vi "climber_globals.vi"() -> ()   [LabVIEW 2020]
panel:
  in  "Climber Traversal Piston Command":bool
  out "Climber Lower Command":bool
  out "Climber Raise Command":bool
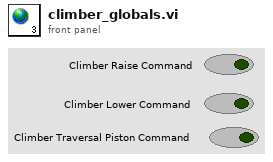
[diagram p1: front panel]
diagram:
